vi "GetCompressionTypes.vi"(7 "force CVT update":bool, 8 "error in":errorcluster, 11 "variable":string) -> (0 "error out":errorcluster, 1 "non compressed":bool, 2 "compressed":bool, 3 "variable out":string, 5 "force CVT update out":bool)   [LabVIEW 2011]
uses:
  FGV_Control.ctl
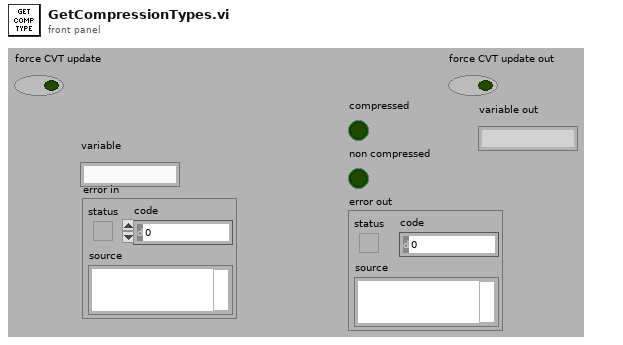
[diagram p1: front panel]
types:
  T1 = typedef "FGV_Control.ctl" = enum16{"add connection", "remove connection", "read variable data", "read connection data", "return all connections", "return all variables", "reset"}
  T2 = typedef "variabledata_typdef.ctl" = cluster{"type":string, "connections (ID)":string, "compressed":bool, "non compressed":bool}
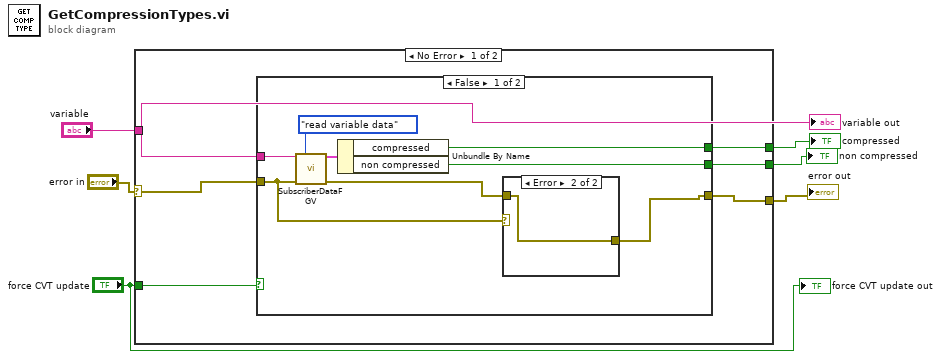
[diagram p0: block diagram]
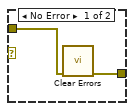
[diagram p2: hidden frame]
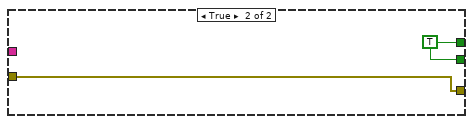
[diagram p3: hidden frame]
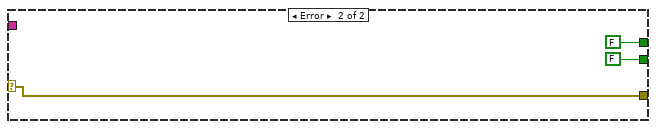
[diagram p4: hidden frame]
diagram:
  n1 = case shown="No Error" "error in" {
    selector: "error in" -> [w8 w28]
    tunnel: "variable" -> [w12 _]
    tunnel: [w11 FALSE ("compressed")] -> w5
    tunnel: [w10 FALSE ("non compressed")] -> w4
    tunnel: [w9 w28] -> w3
    tunnel: "force CVT update" -> [w7 _]
    frame No Error {
      n2 = case shown="False" w7 {
        tunnel: w12 -> [w20 _]
        tunnel: [w19 w25] -> w11
        tunnel: [w18 w25] -> w10
        tunnel: [w14 w24] -> w9
        tunnel: w8 -> [w13 w24]
        frame False {
          n3 = call "SubscriberDataFGV.vi"("variable"=w20, "command"=FGV_Control."read variable data", "error in (no error)"=w13) -> ("variable data"=w16:T2, "error out"=w15:errorcluster)  [unwired: 8 in, 3 out]
          n4 = Unbundle By Name(w16) -> ("compressed"=w19:bool, "non compressed"=w18:bool)
          n5 = case shown="Error" w13 {
            tunnel: w15 -> [w22 w23]
            tunnel: [w21 w23] -> w14
            frame No Error {
              n6 = call "Clear Errors.vi"("error in (no error)"=w22) -> ("error out"=w21:errorcluster)  [unwired: 6 in]
            }
            frame Error {
            }
          }
        }
        frame True {
          w25 = TRUE ("compressed")
        }
      }
    }
    frame Error {
    }
  }
  "compressed" <- w5
  "non compressed" <- w4
  "error out" <- w3
  "force CVT update out" <- "force CVT update"
  "variable out" <- "variable"
